vi "MGI Union and Intersection.vi"(10 "Sequence 2[]":string[](array[string]), 11 "Sequence 1[]":string[](array[string])) -> (0 "Union[]":string[](array[string]), 1 "Intersection[]":string[](array[string]), 2 "Unique Values 2[]":string[](array[string]), 3 "Unique Values 1[]":string[](array[string]))   [LabVIEW 2020]
doc: "Given the two ordered sequences, find the Union containing all values, the Intersection containing values in both sequences, and the values unique to each sequence. All arrays maintain the order of the orginal sequences. If elements appear in a different order in the sequences, the first sequence takes precedence.\nNote: \"ordered\" does not necessarily mean alphabetical.\nNote: Duplicates in Sequence 1 or Sequence 2 are removed in the output arrays.\n\nAuthored by Shawn Walpole\nsupport@mooregoodideas.com\nwww.mooregoodideas.com\n\nCopyright (c) 2010, Moore Good Ideas, Inc.\n\nAll rights reserved.\n\nRedistribution and use in source and binary forms, with or without modification, are permitted provided that the following conditions are met:\n\n * Redistributions of source code must retain the above copyright notice, this list of conditions and the following disclaimer.\n * Redistributions in binary form must reproduce the above copyright notice, this list of conditions and the following disclaimer in the documentation and/or other materials provided with the distribution.\n * Neither the name of Moore Good Ideas, Inc. nor the names of its contributors may be used to endorse or promote products derived from this software without specific prior written permission.\n\nTHIS SOFTWARE IS PROVIDED BY THE COPYRIGHT HOLDERS AND CONTRIBUTORS \"AS IS\" AND ANY EXPRESS OR IMPLIED WARRANTIES, INCLUDING, BUT NOT LIMITED TO, THE IMPLIED WARRANTIES OF MERCHANTABILITY AND FITNESS FOR A PARTICULAR PURPOSE ARE DISCLAIMED. IN NO EVENT SHALL THE COPYRIGHT OWNER OR CONTRIBUTORS BE LIABLE FOR ANY DIRECT, INDIRECT, INCIDENTAL, SPECIAL, EXEMPLARY, OR CONSEQUENTIAL DAMAGES (INCLUDING, BUT NOT LIMITED TO, PROCUREMENT OF SUBSTITUTE GOODS OR SERVICES; LOSS OF USE, DATA, OR PROFITS; OR BUSINESS INTERRUPTION) HOWEVER CAUSED AND ON ANY THEORY OF LIABILITY, WHETHER IN CONTRACT, STRICT LIABILITY, OR TORT (INCLUDING NEGLIGENCE OR OTHERWISE) ARISING IN ANY WAY OUT OF THE USE OF THIS SOFTWARE, EVEN IF ADVISED OF THE POSSIBILITY OF SUCH DAMAGE."
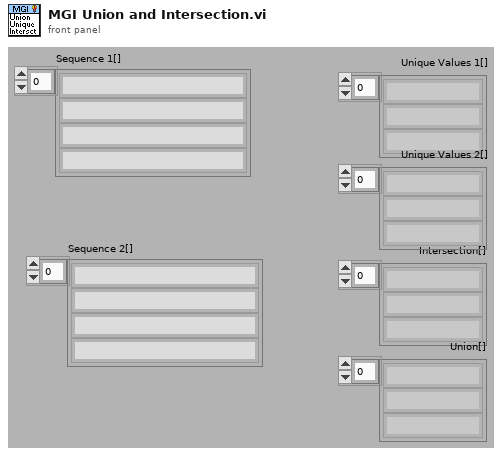
[diagram p1: front panel]
types:
  T1 = cluster{bool, "Seq1 Idx":i32, "Seq2 Idx":i32, i32}
  T2 = cluster{bool, bool, bool, "Seq1 Idx":i32, "Seq2 Idx":i32, i32}
  T3 = cluster{bool, bool, bool, "Seq1 Idx":i32, "Seq2 Idx":i32, i32}[]
  T4 = cluster{bool, "Seq1 Idx":i32, "Seq2 Idx":i32, i32}[]
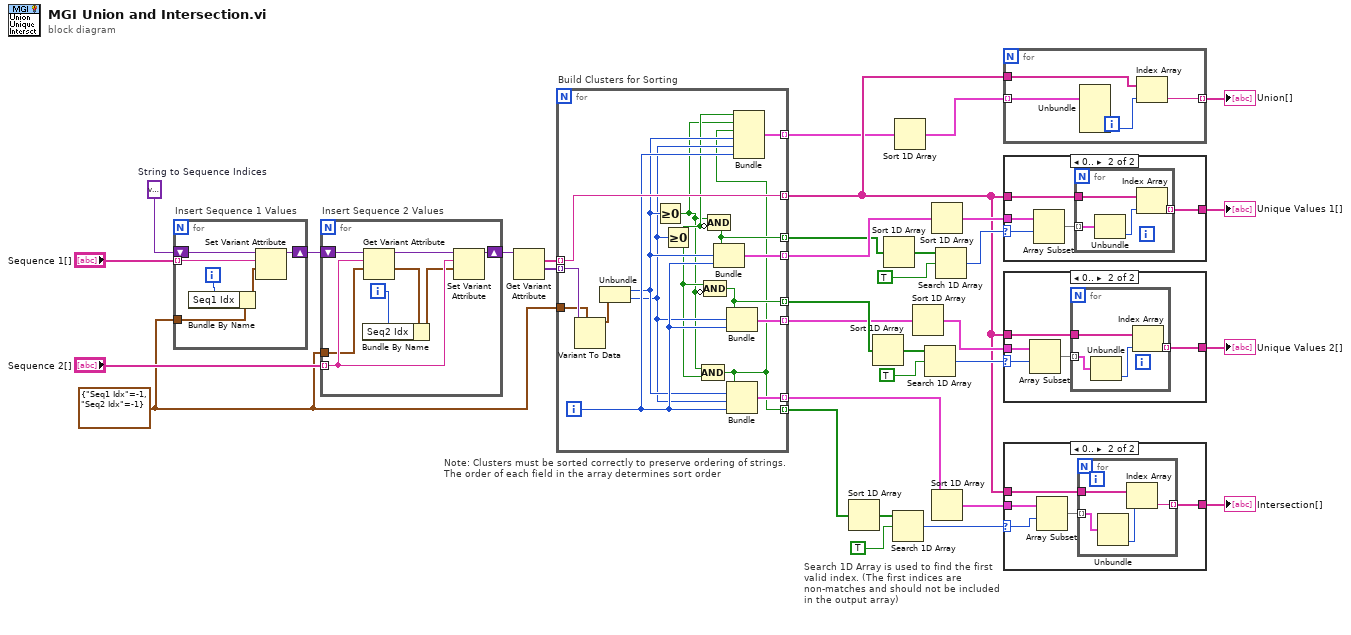
[diagram p0: block diagram]
diagram:
  w1 = cluster{"Seq1 Idx":i32, "Seq2 Idx":i32} {"Seq1 Idx"=-1, "Seq2 Idx"=-1} ("cluster")
  w33 = variant  # String to Sequence Indices
  # "Search 1D Array is used to find the first valid index. (The first indices are non-matches and should not be included in the output array)"
  # "Note: Clusters must be sorted correctly to preserve ordering of strings.\nThe order of each field in the array determines sort order"
  n1 = for "Insert Sequence 1 Values" {
    shift-right: [w38] -> w31
    shift-left: w33 -> [w39]
    tunnel: "Sequence 1[]" -> [w37] mode=indexing
    tunnel: w1 -> [w36]
    i -> [w35]
    n2 = Bundle By Name(cluster=w36, "Seq1 Idx"=w35) -> (w34:cluster{"Seq1 Idx":i32, "Seq2 Idx":i32})
    n3 = Set Variant Attribute(Variant=w39, name=w37, value=w34) -> (Variant out=w38:variant)  [unwired: 1 in, 2 out]
  }
  n4 = for "Insert Sequence 2 Values" {
    shift-right: [w47] -> w29
    shift-left: w31 -> [w46]
    tunnel: "Sequence 2[]" -> [w45] mode=indexing
    tunnel: w1 -> [w43]
    i -> [w42]
    n5 = Get Variant Attribute(Variant=w46, name=w45, default value (empty Variant)=w43) -> (duplicate Variant=w44:variant, value=w40:cluster{"Seq1 Idx":i32, "Seq2 Idx":i32})  [unwired: 1 in, 2 out]
    n6 = Bundle By Name(cluster=w40, "Seq2 Idx"=w42) -> (w41:cluster{"Seq1 Idx":i32, "Seq2 Idx":i32})
    n7 = Set Variant Attribute(Variant=w44, name=w45, value=w41) -> (Variant out=w47:variant)  [unwired: 1 in, 2 out]
  }
  n8 = Get Variant Attribute(Variant=w29) -> (names=w28:string[], values=w27:variant[])  [unwired: 3 in, 2 out]
  n9 = for "Build Clusters for Sorting" {
    tunnel: w28 -> [w59] mode=indexing
    tunnel: w27 -> [w63] mode=indexing
    tunnel: w1 -> [w62]
    tunnel: [w60] -> w10 mode=indexing
    tunnel: [w59] -> w5 mode=indexing
    tunnel: [w58] -> w13 mode=indexing
    tunnel: [w57] -> w26 mode=indexing
    tunnel: [w50] -> w25 mode=indexing
    tunnel: [w55] -> w9 mode=indexing
    tunnel: [w56] -> w14 mode=indexing
    tunnel: [w53] -> w4 mode=indexing
    i -> [w54]
    n10 = Variant To Data(type=w62, Variant=w63) -> (data=w61:cluster{"Seq1 Idx":i32, "Seq2 Idx":i32})  [unwired: 1 in, 1 out]
    n11 = Unbundle(w61) -> ("Seq1 Idx"=w52:i32, "Seq2 Idx"=w51:i32)
    n12 = Greater Or Equal To 0?(x=w52) -> (x >= 0?=w48:bool)
    n13 = Greater Or Equal To 0?(x=w51) -> (x >= 0?=w49:bool)
    n14 = Compound Arithmetic op=AND(w48, w49) -> (w50:bool)
    n15 = Compound Arithmetic op=AND(w49, invert w48) -> (w56:bool)
    n16 = Compound Arithmetic op=AND(w48, invert w49) -> (w55:bool)
    n17 = Bundle(w55, "Seq1 Idx"=w52, w54) -> (w60:cluster{bool, "Seq1 Idx":i32, i32})  [unwired: 1 in]
    n18 = Bundle(w56, "Seq2 Idx"=w51, w54) -> (w58:cluster{bool, "Seq2 Idx":i32, i32})  [unwired: 1 in]
    n19 = Bundle(w50, "Seq1 Idx"=w52, "Seq2 Idx"=w51, w54) -> (w57:T1)  [unwired: 1 in]
    n20 = Bundle(w49, w48, w50, "Seq1 Idx"=w52, "Seq2 Idx"=w51, w54) -> (w53:T2)  [unwired: 1 in]
  }
  n21 = Sort 1D Array(array=w25) -> (sorted array=w24:bool[])
  n22 = Sort 1D Array(array=w14) -> (sorted array=w17:bool[])
  n23 = Sort 1D Array(array=w9) -> (sorted array=w12:bool[])
  n24 = Search 1D Array(1D array=w24, element=TRUE) -> (index of element=w21:i32)  [unwired: 1 in]
  n25 = Sort 1D Array(array=w4) -> (sorted array=w3:T3)
  n26 = Sort 1D Array(array=w13) -> (sorted array=w15:cluster{bool, "Seq2 Idx":i32, i32}[])
  n27 = Search 1D Array(1D array=w17, element=TRUE) -> (index of element=w16:i32)  [unwired: 1 in]
  n28 = Sort 1D Array(array=w10) -> (sorted array=w7:cluster{bool, "Seq1 Idx":i32, i32}[])
  n29 = Sort 1D Array(array=w26) -> (sorted array=w22:T4)
  n30 = Search 1D Array(1D array=w12, element=TRUE) -> (index of element=w8:i32)  [unwired: 1 in]
  n31 = for {
    tunnel: w3 -> [w65] mode=indexing
    tunnel: w5 -> [w67]
    tunnel: [w66] -> w2 mode=indexing
    n32 = Unbundle(w65) -> (w64:i32)  [unwired: 5 out]
    n33 = Index Array(array=w67, index=w64) -> (element=w66:string)
  }
  "Union[]" <- w2
  n34 = case shown="0.." w8 {
    selector: w8 -> [_ w69]
    tunnel: w5 -> [_ w72]
    tunnel: w7 -> [_ w71]
    tunnel: [_ w68] -> w6
    frame ..-1 {
    }
    frame 0.. {
      n35 = Array Subset(array=w71, index=w69) -> (w70:cluster{bool, "Seq1 Idx":i32, i32}[])  [unwired: 1 in]
      n36 = for {
        tunnel: w70 -> [w76] mode=indexing
        tunnel: w72 -> [w75]
        tunnel: [w74] -> w68 mode=indexing
        n37 = Unbundle(w76) -> (w73:i32)  [unwired: 2 out]
        n38 = Index Array(array=w75, index=w73) -> (element=w74:string)
      }
    }
  }
  "Unique Values 1[]" <- w6
  n39 = case shown="0.." w16 {
    selector: w16 -> [_ w78]
    tunnel: w5 -> [_ w81]
    tunnel: w15 -> [_ w80]
    tunnel: [_ w77] -> w19
    frame ..-1 {
    }
    frame 0.. {
      n40 = Array Subset(array=w80, index=w78) -> (w79:cluster{bool, "Seq2 Idx":i32, i32}[])  [unwired: 1 in]
      n41 = for {
        tunnel: w79 -> [w85] mode=indexing
        tunnel: w81 -> [w84]
        tunnel: [w83] -> w77 mode=indexing
        n42 = Unbundle(w85) -> (w82:i32)  [unwired: 2 out]
        n43 = Index Array(array=w84, index=w82) -> (element=w83:string)
      }
    }
  }
  "Unique Values 2[]" <- w19
  n44 = case shown="0.." w21 {
    selector: w21 -> [_ w87]
    tunnel: w5 -> [_ w90]
    tunnel: w22 -> [_ w89]
    tunnel: [_ w86] -> w20
    frame ..-1 {
    }
    frame 0.. {
      n45 = Array Subset(array=w89, index=w87) -> (w88:T4)  [unwired: 1 in]
      n46 = for {
        tunnel: w88 -> [w94] mode=indexing
        tunnel: w90 -> [w93]
        tunnel: [w92] -> w86 mode=indexing
        n47 = Unbundle(w94) -> (w91:i32)  [unwired: 3 out]
        n48 = Index Array(array=w93, index=w91) -> (element=w92:string)
      }
    }
  }
  "Intersection[]" <- w20
